vi "SubTemplate_4x4x4_Delete.vi"(8 "error in (no error)":errorcluster, 10 "Force delete":bool, 11 "reference in":refnum<class "SubTemplate_4x4x4.lvclass">) -> (0 "error out":errorcluster, 2 "# of objects":i32, 3 "reference out":refnum<class "SubTemplate_4x4x4.lvclass">)   [LabVIEW 2016, in "SubTemplate_4x4x4.lvclass"]
doc: "Deletes an object created with this class new VI and returns the contents of the object."
uses:
  <resource>/Framework/Providers/Open_GDS/ClassProviders/Provider_EndevoGOOP300/Templates/SubTemplate_4x4x4/SubTemplate_4x4x4.lvclass
  <vilib>/addons/_goop3.llb/3GOOPStates.ctl
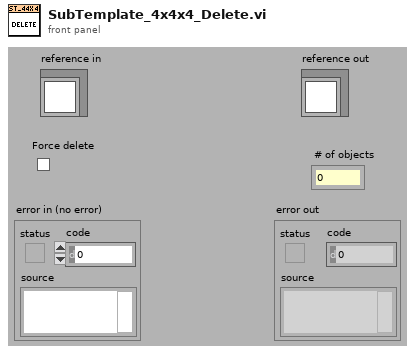
[diagram p1: front panel]
types:
  T1 = typedef "3GOOPStates.ctl" = enum16{"Set", "Get", "New", "Delete", "Clear", "Test and get", "Unlock data", "Information", "Look up existing", "New or look up existing", "Test and get shared", "Get shared", "Set shared", "Unlock shared", "Find dynamic method", "Register dynamic method", "Preload dynamic method", "Probe", "Cast to more generic", "Cast to more specific"}
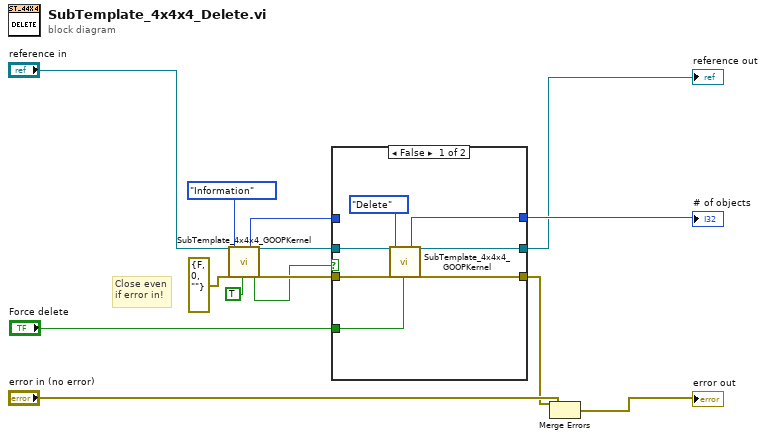
[diagram p0: block diagram]
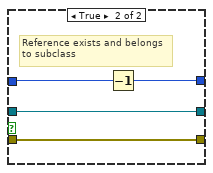
[diagram p2: hidden frame]
diagram:
  # "Close even\nif error in!"
  n1 = call <resource>:"SubTemplate_4x4x4_GOOPKernel.vi"("Ref in"="reference in", "error in (no error)"=errorcluster {"status"=FALSE, "code"=0, "source"=""}, "Action"=3GOOPStates."Information", "Misc"=TRUE) -> ("# of objects"=w8:i32, "IsSubclass?"=w2:bool, "Ref out"=w10:refnum<class "SubTemplate_4x4x4.lvclass">, "error out"=w11:errorcluster)  [unwired: 13 in, 7 out]
  n2 = case shown="False" w2 {
    tunnel: [w21 w23] -> w12
    tunnel: [w18 w25] -> w6
    tunnel: w11 -> [w20 w23]
    tunnel: w10 -> [w19 w22]
    tunnel: w8 -> [_ w24]
    tunnel: [w16 w22] -> w3
    tunnel: "Force delete" -> [w15 _]
    frame False {
      n3 = call <resource>:"SubTemplate_4x4x4_GOOPKernel.vi"("Ref in"=w19, "error in (no error)"=w20, "Action"=3GOOPStates."Delete", "Misc"=w15) -> ("# of objects"=w18:i32, "Ref out"=w16:refnum<class "SubTemplate_4x4x4.lvclass">, "error out"=w21:errorcluster)  [unwired: 13 in, 8 out]
    }
    frame True {
      # "Reference exists and belongs\nto subclass"
      n4 = Decrement(x=w24) -> (x-1=w25:i32)
    }
  }
  "reference out" <- w3
  "# of objects" <- w6
  n5 = Merge Errors("error in (no error)", w12) -> (→"error out":errorcluster)
